vi "AlazarGetCPLDVersion.vi"(0 "Handle":u64, 11 "error in (no error)":errorcluster) -> (4 "Handle":u64, 6 "Major":u8, 8 "Minor":u8, 10 "Return Code":u32, 15 "error out":errorcluster)   [LabVIEW 2018]
doc: "Get the CPLD version number of the specified board."
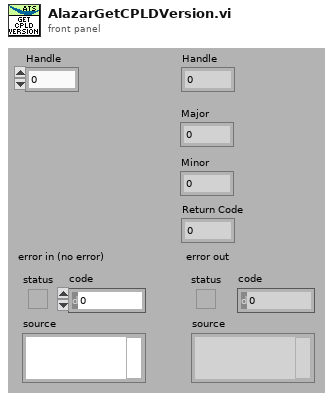
[diagram p1: front panel]
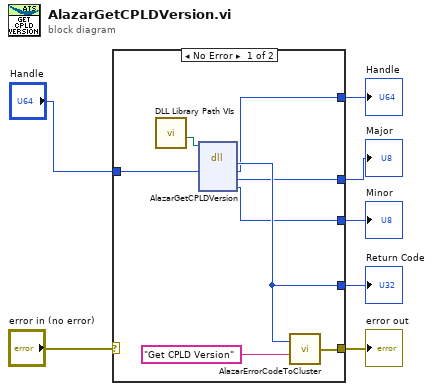
[diagram p0: block diagram]
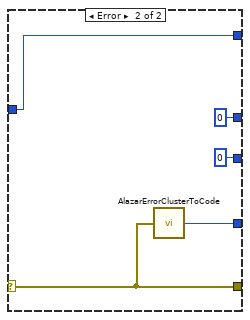
[diagram p2: hidden frame]
diagram:
  n1 = case shown="No Error" "error in (no error)" {
    selector: "error in (no error)" -> [_ w20]
    tunnel: [w12 w20] -> w6
    tunnel: [w14 w19] -> w5
    tunnel: "Handle" -> [w15 w18]
    tunnel: [w11 w18] -> w3
    tunnel: [w10 0] -> w2
    tunnel: [w9 0] -> w1
    frame No Error {
      n2 = call "DLL Library Path VIs.vi"() -> ("Alazar"=w8:path)  [unwired: 9 in, 2 out]
      n3 = dll-call lib="C:/Project/SerialSectOCT - FFT GPU/SerialSectOCT/Labview Software/DLL/ATSApi.dll" fn="AlazarGetCPLDVersion"(path in=w8, "handle"=w15) -> ("return type"=w14:u32, "handle"=w11:u64, "major"=w10:u8, "minor"=w9:u8)  [unwired: 4 in, 2 out]
      n4 = call "AlazarErrorCodeToCluster.vi"("Message"="Get CPLD Version", "Error Code"=w14) -> ("error out"=w12:errorcluster)
    }
    frame Error {
      n5 = call "AlazarErrorClusterToCode.vi"("error in (no error)"=w20) -> ("Error Code"=w19:u32)
    }
  }
  "Handle" <- w3
  "error out" <- w6
  "Return Code" <- w5
  "Minor" <- w1
  "Major" <- w2
